vi "About ProSCI.vi"() -> ()   [LabVIEW 2012]
panel:
  in  "?":bool
  # "ProSCI"
  # "3.1 (Beta)"
  # "Programmable Sectioning & Cryo-Imaging"
  # "bme.case.edu/bmil"
  # "ProSCI © 2006-07 Case BME Imaging Lab"
  # "Labview © 2006 National Instruments"
  # "Debashish.Roy@case.edu"
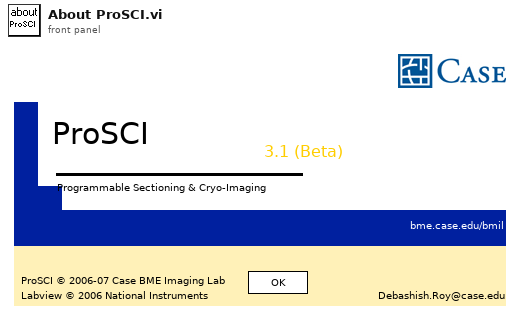
[diagram p1: front panel]
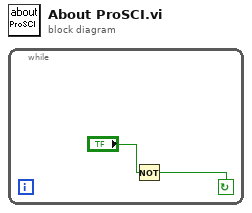
[diagram p0: block diagram]
diagram:
  n1 = while {
    stop <- w1 continue-if-true
    n2 = Not(x="?") -> (.not. x?=w1:bool)
  }
